vi "Record.vi"(8 "error in (no error)":errorcluster, 10 "Record State":u16(ring) items=["ON", "OFF", "TRIG"], 11 "VISA resource name":refnum<visa-resource-name>) -> (0 "error out":errorcluster, 3 "VISA resource name out":refnum<visa-resource-name>)   [LabVIEW 2017, in "Sefram DAS220.lvlib"]
doc: "Start, stop or force the record to start an acquisition into internal memory."
uses:
  <instrlib>/Sefram DAS220/Sefram DAS220.lvlib
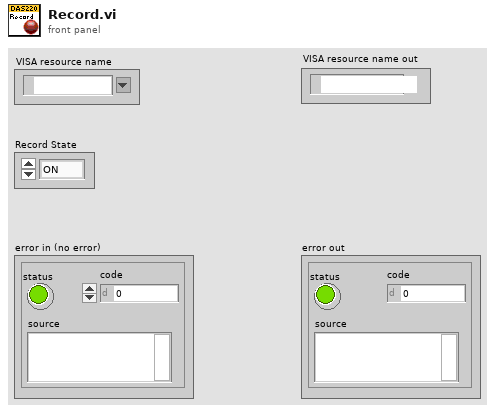
[diagram p1: front panel]
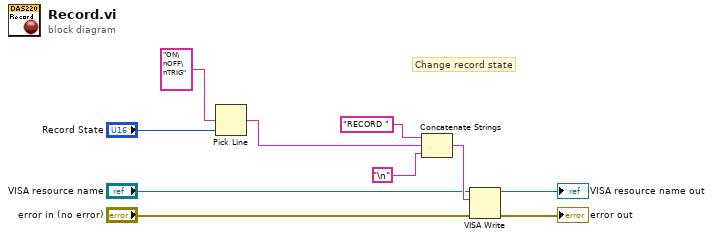
[diagram p0: block diagram]
diagram:
  # "Change record state"
  n1 = Pick Line(multi-line string="ON\nOFF\nTRIG", line index="Record State") -> (output string=w2:string)  [unwired: 1 in]
  n2 = Concatenate Strings("RECORD " ("string"), w2, "\n") -> (w10:string)
  n3 = VISA Write(VISA resource name="VISA resource name", write buffer=w10, error in (no error)="error in (no error)") -> (VISA resource name out=→"VISA resource name out":refnum<visa-resource-name>, error out=→"error out":errorcluster)  [unwired: 1 out]
